vi "Music Visualizer (Queue Only).vi"(11 "Mixed Audio Data":refnum<queue>) -> ()   [LabVIEW 2020]
doc: "A simple music visualizer.\n\nDemonstrates the G-Audio mixer and the mixed audio queue feature."
uses:
  <vilib>/Analysis/1siggen.llb/Ramp Pattern by Samples.vi
  <vilib>/Analysis/5stat.llb/RMS (DBL).vi
  <vilib>/Analysis/NI_AALPro.lvlib
  <vilib>/ptbypt/NI_PtbyPt.lvlib
  <vilib>/Analysis/NI_AALBase.lvlib
panel:
  in  "Size":dbl(slide)=1.0 scale=0.5..1.5
  in  "Color Box":u32(colorbox)=5883391
  in  "Close":bool
  out "XY Graph":cluster{dbl[], dbl[]}[](graph)
  # "+"
  # "-"
  # "Instructions:\n1. Trigger playback in the main Sample Pad window."
  # "G"
  # "-Audio"
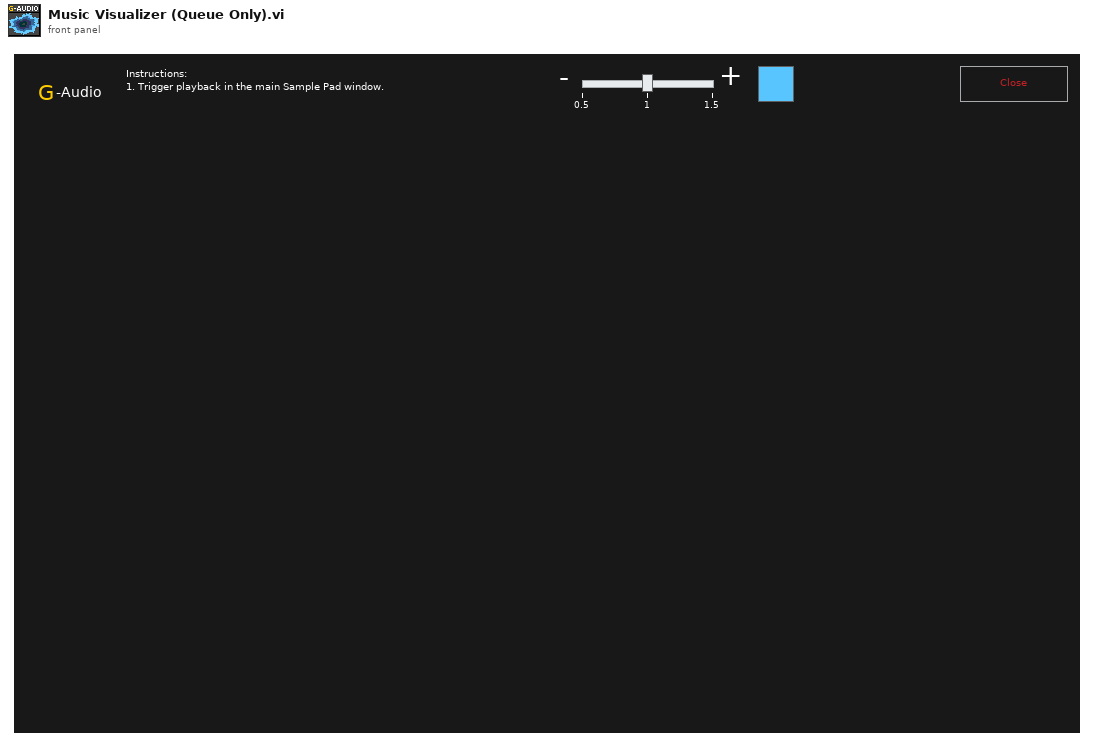
[diagram p1: front panel]
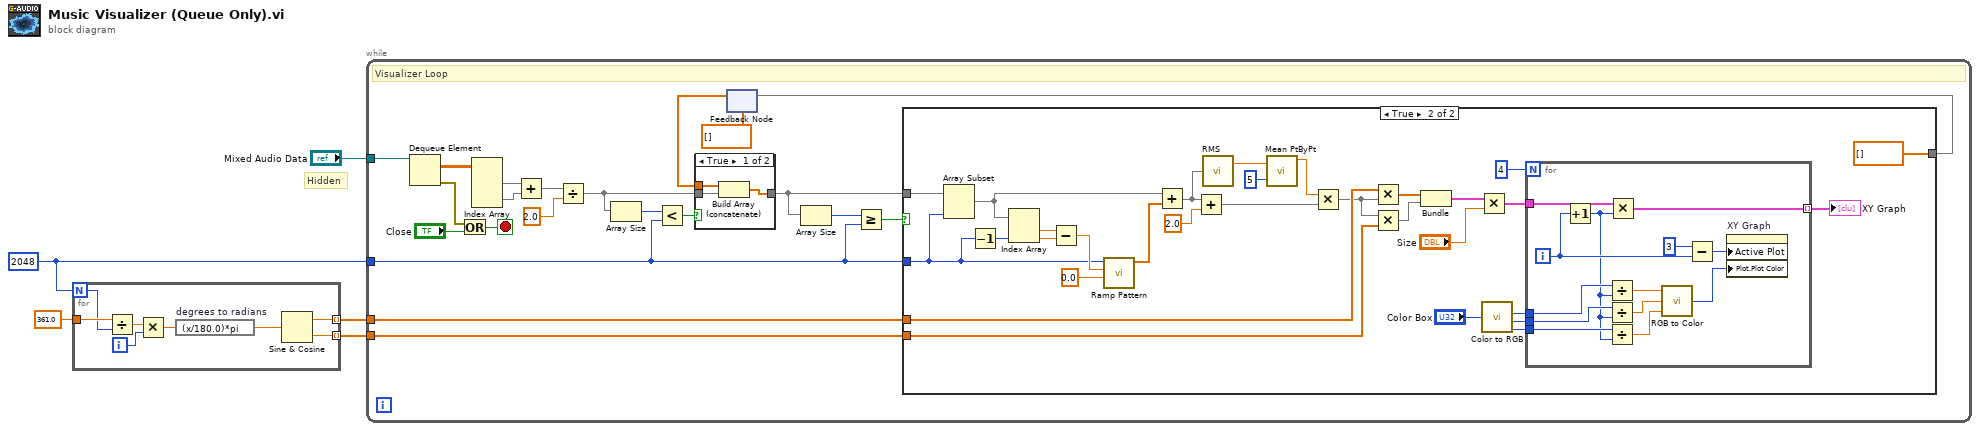
[diagram p0: block diagram]
diagram:
  w1 = 2048 ("Buffer Size (samples)")
  # "Hidden"
  n1 = for {
    N: w1 -> [w12]
    tunnel: 361.0 -> [w13]
    tunnel: [w8] -> w4 mode=indexing
    tunnel: [w7] -> w3 mode=indexing
    i -> [w10]
    n2 = Divide(x=w13, y=w12) -> (x/y=w11:dbl)
    n3 = Multiply(x=w11, y=w10) -> (x*y=w9:dbl)
    n4 = expression code="(x/180.0)*pi" "degrees to radians"(w9) -> (w6:dbl)
    n5 = Sine & Cosine(0:w6) -> (1:w8:dbl, 2:w7:dbl)
  }
  n6 = while {
    tunnel: w4 -> [w34]
    tunnel: w3 -> [w33]
    tunnel: "Mixed Audio Data" -> [w32]
    tunnel: w1 -> [w22]
    stop <- w30 stop-if-true
    # "Visualizer Loop"
    n7 = Dequeue Element(queue=w32) -> (element=w19:dbl[][], error out=w31:errorcluster)  [unwired: 2 in, 2 out]
    n8 = Or(x=w31, y="Close") -> (x .or. y?=w30:bool)
    n9 = Index Array(array=w19) -> (element #1=w18:dbl[], element #2=w17:dbl[])  [unwired: 4 in]
    n10 = Add(x=w18, y=w17) -> (x+y=w16:dbl[])
    n11 = Divide(x=w16, y=2.0) -> (x/y=w15:dbl[])
    n12 = Array Size(array=w15) -> (size(s)=w28:i32)
    n13 = Less?(x=w28, y=w22) -> (x < y?=w27:bool)
    n14 = feedback #1(dbl[] [] ("Audio Data")) -> (w26:dbl[])
    n15 = case shown="True" w27 {
      tunnel: w15 -> [w81 w82]
      tunnel: [w80 w82] -> w23
      tunnel: w26 -> [w79 _]
      frame True {
        n16 = Build Array (concatenate)(w79, w81) -> (w80:dbl[])
      }
      frame False {
      }
    }
    n17 = Array Size(array=w23) -> (size(s)=w25:i32)
    n18 = Greater Or Equal?(x=w25, y=w22) -> (x >= y?=w24:bool)
    n19 = case shown="True" w24 {
      tunnel: w34 -> [_ w65]
      tunnel: w33 -> [_ w64]
      tunnel: w23 -> [w35 w39]
      tunnel: w22 -> [_ w37]
      tunnel: [w35 dbl[] [] ("Audio Data")] -> w21
      frame False {
      }
      frame True {
        n20 = Array Subset(array=w39, length=w37) -> (w38:dbl[])  [unwired: 1 in]
        n21 = Decrement(x=w37) -> (x-1=w49:i32)
        n22 = Index Array(array=w38, index #2=w49) -> (element #1=w44:dbl, element #2=w45:dbl)  [unwired: 1 in]
        n23 = Subtract(x=w44, y=w45) -> (x-y=w46:dbl)
        n24 = call-poly <vilib>:"Ramp Pattern.vi"("start"=0.0, "end"=w46, "samples"=w37) -> ("Ramp Pattern"=w48:dbl[])  [unwired: 7 in, 1 out]
        n25 = Add(x=w38, y=w48) -> (x+y=w43:dbl[])
        n26 = Add(x=w43, y=2.0) -> (x+y=w63:dbl[])
        n27 = call-poly <vilib>:"RMS.vi"("X"=w43) -> ("rms value"=w52:dbl)  [unwired: 1 out]
        n28 = call <vilib>:"Mean PtByPt.vi"("x"=w52, "sample length"=5) -> ("mean"=w51:dbl)  [unwired: 2 in, 1 out]
        n29 = Multiply(x=w51, y=w63) -> (x*y=w53:dbl[])
        n30 = Multiply(x=w65, y=w53) -> (x*y=w61:dbl[])
        n31 = Multiply(x=w53, y=w64) -> (x*y=w60:dbl[])
        n32 = Bundle(w61, w60) -> (w41:cluster{dbl[], dbl[]})  [unwired: 1 in]
        n33 = Multiply(x=w41, y="Size") -> (x*y=w40:cluster{dbl[], dbl[]})
        n34 = call <vilib>:"Color to RGB.vi"("Color"="Color Box") -> ("R"=w56:u8, "G"=w55:u8, "B"=w54:u8)  [unwired: 1 out]
        n35 = for {
          N: 4 -> [_]
          tunnel: w40 -> [w78]
          tunnel: [w77] -> w58 mode=indexing
          tunnel: w56 -> [w75]
          tunnel: w55 -> [w74]
          tunnel: w54 -> [w73]
          i -> [w76]
          n36 = Increment(x=w76) -> (x+1=w72:i32)
          n37 = Divide(x=w75, y=w72) -> (x/y=w69:dbl)
          n38 = Divide(x=w74, y=w72) -> (x/y=w68:dbl)
          n39 = Divide(x=w73, y=w72) -> (x/y=w71:dbl)
          n40 = Multiply(x=w78, y=w72) -> (x*y=w77:cluster{dbl[], dbl[]})
          n41 = call <vilib>:"RGB to Color.vi"("B"=w71, "G"=w68, "R"=w69) -> ("Color"=w70:u32)
          n42 = Subtract(x=3, y=w76) -> (x-y=w67:i32)
          n43 = property on="XY Graph" class="XYGraph (strict)"("Active Plot"=w67, "Plot.Plot Color"=w70) -> ()  [unwired: 2 in, 2 out]
        }
        "XY Graph" <- w58
      }
    }
    n44 = feedback-in #1(w21) -> ()
  }
